vi "SetCtlValue.vi"(8 "Error in":errorcluster, 9 "Value":variant, 10 "CtlName In":string, 11 "CtlLookup In":T1) -> (0 "error out":errorcluster, 3 "CtlLookup Out":T1)   [LabVIEW 2020, in "CtlReferences.lvlib" / "CtlReferences.lvclass"]
uses:
  CtlReferences.lvclass
  CtlReferences.lvclass/CtlReferences.ctl
  TypeDefs/CtlLookup.ctl
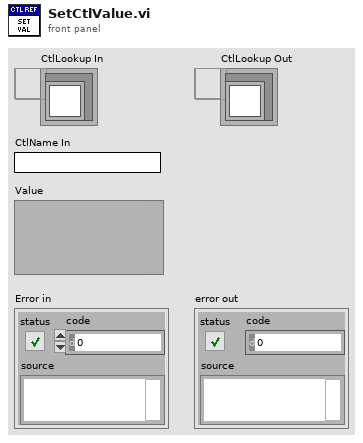
[diagram p1: front panel]
types:
  T1 = typedef "CtlReferences.lvlib/CtlReferences.lvclass/CtlLookup.ctl" = refnum<data-value>
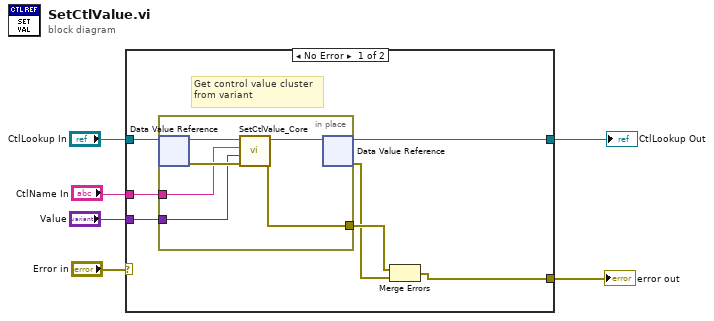
[diagram p0: block diagram]
diagram:
  n1 = case shown="No Error" "Error in" {
    selector: "Error in" -> [_ w21]
    tunnel: [w13 w20] -> w6
    tunnel: "CtlName In" -> [w8 _]
    tunnel: "CtlLookup In" -> [w12 w20]
    tunnel: [w11 w21] -> w3
    tunnel: "Value" -> [w7 _]
    frame No Error {
      # "Get control value cluster\nfrom variant"
      n2 = in-place {
        in-place-border: [w18] -> w10
        in-place-border: w8 -> [w15]
        in-place-border: w7 -> [w14]
        n3 = in-place-dvr #1(w12) -> (w17:refnum<class "CtlReferences.lvclass">, w19:errorcluster)
        n4 = call-dynamic "SetCtlValue_Core.vi"("error in (no error)"=w19, "Value"=w14, "CtlName In"=w15, "CtlReferences in"=w17) -> ("error out"=w18:errorcluster, "CtlReferences out"=w16:refnum<class "CtlReferences.lvclass">)  [unwired: 6 in]
        n5 = in-place-dvr #1(w16) -> (w13:T1, w9:errorcluster)
      }
      n6 = Merge Errors(w10, w9) -> (w11:errorcluster)
    }
    frame Error {
    }
  }
  "error out" <- w3
  "CtlLookup Out" <- w6
